vi "Configure Output Delay.vi"(0 "VISA resource name":refnum<visa-resource-name>, 1 "Delay Type":u16(ring) items=["On", "Off", "Rise", "Fall"], 2 "Delay(S)":dbl min=0.0 max=10.0 step=0.001, 3 "error in":errorcluster) -> (7 "VISA resource name out":refnum<visa-resource-name>, 10 "error out":errorcluster)   [LabVIEW 2018, in "IT-M3100.lvlib"]
doc: "This command sets the delay time.\n<b>Delay Type</b>\n0:On :This command sets the delay time before turning the output on.\n1:Off :This command sets the delay time after turning the output off.\n2:Rise :This command sets the delay time before turning the output on.\n3:Fall :This command sets the delay time after turning the output off.\n<b>Delay(S)</b>\n0-10"
uses:
  IT-M3100.lvlib
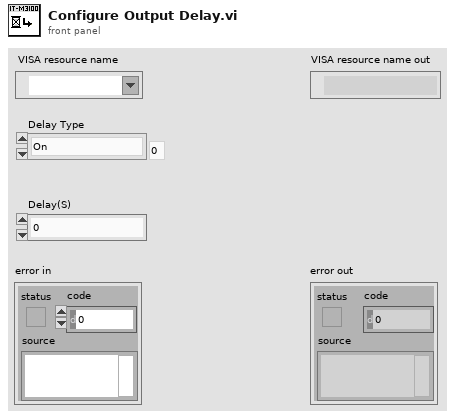
[diagram p1: front panel]
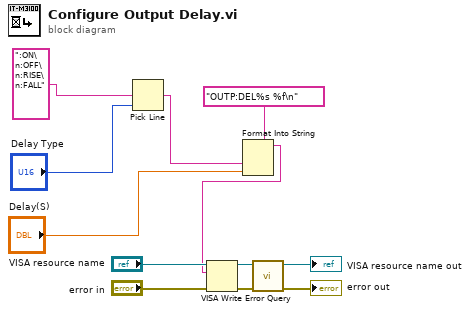
[diagram p0: block diagram]
diagram:
  n1 = Pick Line(multi-line string=":ON\n:OFF\n:RISE\n:FALL", line index="Delay Type") -> (output string=w2:string)  [unwired: 1 in]
  n2 = Format Into String(format string="OUTP:DEL%s %f\n", w2, "Delay(S)") -> (resulting string=w1:string)  [unwired: 2 in, 1 out]
  n3 = VISA Write(VISA resource name="VISA resource name", write buffer=w1, error in (no error)="error in") -> (VISA resource name out=w9:refnum<visa-resource-name>, error out=w10:errorcluster)  [unwired: 1 out]
  n4 = call "Error Query.vi"("error in"=w10, "VISA resource name"=w9) -> ("error out"=→"error out":errorcluster, "VISA resource name out"=→"VISA resource name out":refnum<visa-resource-name>)  [unwired: 6 in, 2 out]
